vi "Create_Serializable_Methods_Path.vi"(8 "error in (no error)":errorcluster, 10 "LVClass library Path":path, 11 "class reference":refnum<vi>) -> (0 "error out":errorcluster)   [LabVIEW 2019, in "BlueSerializationScripts.lvlib"]
uses:
  BlueSerializationScripts.lvlib
  Support/AccessDirection.ctl
  UserAppLibs/IncrementMutationHistory/IncrementBlueSerVersionAction.ctl
  BlueUtilityScripts/BlueUtilityScripts.lvlib
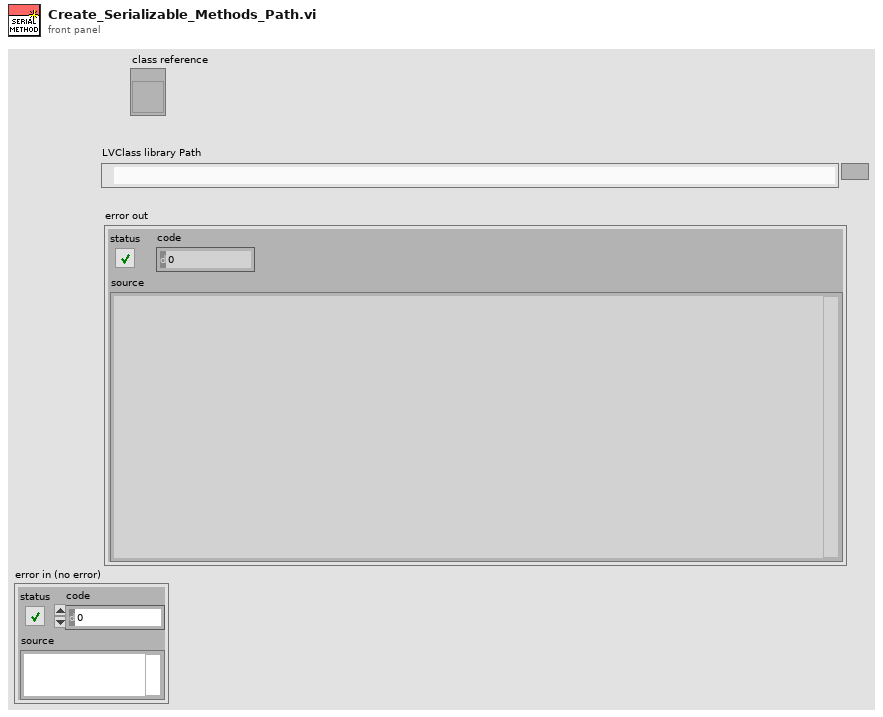
[diagram p1: front panel]
types:
  T1 = typedef "BlueSerializationScripts.lvlib/IncrementBlueSerVersionAction.ctl" = enum16{"Init", "Increment"}
  T2 = typedef "BlueSerializationScripts.lvlib/AccessDirection.ctl" = enum16{"Get", "Set"}
  T3 = typedef "BlueSerializationScripts.lvlib/BlueSerializableTemplatePaths.ctl" = cluster{"GetSerializableData.vi":path, "SerializableData.ctl":path, "SetSerializableData.vi":path, "GetVersionSerializableData.vi":path, "HandleVersionMutation.vi":path, "Mutate_Template.vi":path}
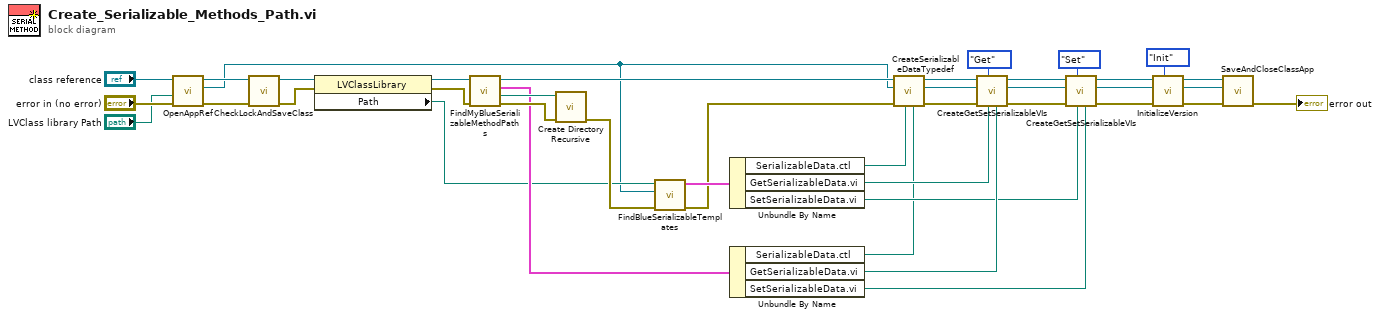
[diagram p0: block diagram]
diagram:
  n1 = call "OpenAppRef.vi"("error in (no error)"="error in (no error)", "LVClass library Path"="LVClass library Path", "class reference"="class reference") -> ("error out"=w15:errorcluster, "Application reference"=w3:refnum<vi>, "LVClass Reference"=w16:refnum<vi>)  [unwired: 6 in]
  n2 = call "CheckLockAndSaveClass.vi"("error in (no error)"=w15, "LVClass ref"=w16) -> ("error out"=w1:errorcluster, "LVClass ref"=w2:refnum<vi>)  [unwired: 8 in]
  n3 = property class="LVClassLibrary"(reference=w2, error in=w1) -> (reference out=w14:refnum<vi>, error out=w13:errorcluster, "Path"=w12:path)
  n4 = call "FindMyBlueSerializableMethodPaths.vi"("error in (no error)"=w13, "LVClass refnum"=w14) -> ("error out"=w36:errorcluster, "BlueSerialization Folder"=w40:path, "BlueSerializable Paths"=w24:T3, "LVClass refnum (dup)"=w20:refnum<vi>)  [unwired: 6 in]
  n5 = call <vilib>:"Create Directory Recursive.vi"("error in (no error)"=w36, "directory"=w40) -> ("error out"=w21:errorcluster)  [unwired: 3 in, 2 out]
  n6 = call "FindBlueSerializableTemplates.vi"("error in (no error)"=w21, "App Reference (this app)"=w3, "LabVIEW Class Path"=w12) -> ("error out"=w32:errorcluster, "BlueSerializableTemplate Paths"=w39:T3)  [unwired: 7 in]
  n7 = Unbundle By Name(w39) -> ("SerializableData.ctl"=w30:path, "GetSerializableData.vi"=w38:path, "SetSerializableData.vi"=w35:path)
  n8 = Unbundle By Name(w24) -> ("SerializableData.ctl"=w29:path, "GetSerializableData.vi"=w37:path, "SetSerializableData.vi"=w34:path)
  n9 = call "CreateSerializableDataTypedef.vi"("SaveTo Path"=w29, "Template typedef path"=w30, "error in (no error)"=w32, "Application"=w3, "LVClassLibrary Ref"=w20) -> ("error out"=w28:errorcluster, "Application"=w31:refnum<vi>, "LVClassLibrary Ref"=w33:refnum<vi>)  [unwired: 4 in]
  n10 = call "CreateGetSetSerializableVIs.vi"("SaveTo Path"=w37, "Template VI path"=w38, "Type"=AccessDirection."Get", "error in (no error)"=w28, "Application"=w31, "LVClassLibrary Ref"=w33) -> ("error out"=w25:errorcluster, "Application"=w26:refnum<vi>, "LVClassLibrary Ref"=w27:refnum<vi>)  [unwired: 3 in]
  n11 = call "CreateGetSetSerializableVIs.vi"("SaveTo Path"=w34, "Template VI path"=w35, "Type"=AccessDirection."Set", "error in (no error)"=w25, "Application"=w26, "LVClassLibrary Ref"=w27) -> ("error out"=w10:errorcluster, "Application"=w8:refnum<vi>, "LVClassLibrary Ref"=w9:refnum<vi>)  [unwired: 3 in]
  n12 = call "InitializeVersion.vi"("Action"=IncrementBlueSerVersionAction."Init", "error in (no error)"=w10, "Application"=w8, "LVClass ref"=w9) -> ("error out"=w5:errorcluster, "Application"=w6:refnum<vi>, "LVClass ref"=w7:refnum<vi>)  [unwired: 4 in, 1 out]
  n13 = call "SaveAndCloseClassApp.vi"("error in (no error)"=w5, "Application"=w6, "LVClassLibrary Ref"=w7) -> ("error out"=→"error out":errorcluster)  [unwired: 8 in]
